vi "PH_Powermeter_BaseClass.contents.vi"   [LabVIEW 2014, in "PH_Powermeter_BaseClass.lvlib"]
doc: "This class is forseen to control a gentec powermeter.\n\nThis class is part of the PHELIX device layer."
uses:
  PH_Powermeter_BaseClass.lvlib
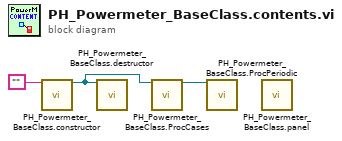
[diagram p0: block diagram]
diagram:
  n1 = call "PH_Powermeter_BaseClass.constructor.vi"("name"="") -> ("i ref out"=w1:refnum<vi>)  [unwired: 16 in, 2 out]
  n2 = call "PH_Powermeter_BaseClass.destructor.vi"("i ref in"=w1) -> ()  [unwired: 18 in, 1 out]
  n3 = call "PH_Powermeter_BaseClass.ProcCases.vi"("i ref in"=w1) -> ("i ref out"=w2:refnum<vi>)  [unwired: 16 in, 2 out]
  n4 = call "PH_Powermeter_BaseClass.ProcPeriodic.vi"("i ref in"=w2) -> ()  [unwired: 16 in, 3 out]
  n5 = call "PH_Powermeter_BaseClass.panel.vi"() -> ()  [unwired: 19 in, 1 out]
